vi "Actor Core.vi"(8 "error in":errorcluster, 11 "ExampleViewManager In":refnum<class "ExampleViewManager.lvclass">) -> (0 "error out":errorcluster, 3 "Actor out":refnum<class "Actor.lvclass">)   [LabVIEW 2017, in "MVA Example.lvlib" / "ExampleViewManager.lvclass"]
doc: "(<B>Filename</B>: Actor Framework.lvlib:Actor.lvclass:Actor Core.vi)\n\nReceives messages to the actor, reacts to them, and initiates any error handling that may shut the actor down.\n\nDescendant classes may override this VI to append parallel tasks for the actor to complete while it handles messages. Overrides use the Call Parent Method node.\n\n<License>\nCopyright © 2017 Composed Systems, LLC | All rights reserved\nwww.composed.io\n\nAuthor: Ethan Stern <ethan.stern@composed.io>\n\nThis software is provided \"AS IS\" WITHOUT WARRANTIES, either express or implied, AND IS FOR EDUCATIONAL PURPOSES ONLY.\n</License>MVA Framework 1.6.0.31\nEthan Stern - Composed Systems\nCopyright (c) 2018, Composed Systems"
uses:
  ExampleViewManager.lvclass
  C:/Program Files (x86)/National Instruments/LabVIEW 2017/vi.lib/Composed Systems/MVA Framework/Framework/ActorEvents/IEventAggregator/IEventAggregator.lvclass
  C:/Program Files (x86)/National Instruments/LabVIEW 2017/vi.lib/ActorFramework/Actor/Actor.lvclass
  <vilib>/ActorFramework/Actor/Actor.lvclass
  <vilib>/event_ctls.llb/lveventtype.ctl
  ExampleViewManager.lvclass/ExampleViewManager.ctl
  <vilib>/ActorFramework/Actor/Actor.lvclass/Actor.ctl
  <vilib>/ActorFramework/Message Enqueuer/Message Enqueuer.lvclass/Message Enqueuer.ctl
  <vilib>/ActorFramework/Report Error Msg/Report Error Msg.lvclass/Report Error Msg.ctl
  <vilib>/ActorFramework/Message Enqueuer/Init from Existing Queue.vi
  <vilib>/ActorFramework/Message Enqueuer/Enqueue.vi
  <vilib>/ActorFramework/Report Error Msg/Report Error Msg.lvclass
  C:/Program Files (x86)/National Instruments/LabVIEW 2017/vi.lib/ActorFramework/Message/Message.lvclass
  <vilib>/ActorFramework/Message Priority Queue/Priority Enqueue.vi
  <vilib>/ActorFramework/Message Enqueuer/Message Enqueuer.lvclass
  <vilib>/Composed Systems/MVA Framework/Framework/IViewManager/IViewManager/IViewManager.lvclass
  MenuButton/MenuButton.lvclass
  MenuButton Event Handler/MenuButton Event Handler.lvclass
  <vilib>/Composed Systems/MVA Framework/Framework/ActorEvents/IEventAggregator/IEventAggregator.lvclass
  <vilib>/Composed Systems/MVA Framework/Framework/IViewable/ProtectedSubpanel/ProtectedSubpanel.lvclass
panel:
  in  "Bool2":bool caption="Blank"
  in  "Main Menu 3":bool caption="Blank"
  in  "Chart2":bool caption="Blank"
  in  "Main Menu 2":bool caption="Blank"
  in  "Slide":bool caption="Blank"
  in  "Listbox":bool caption="Blank"
  in  "Bool1":bool caption="Blank"
  in  "Chart":bool caption="Blank"
  in  "Quad Menu":bool caption="Blank"
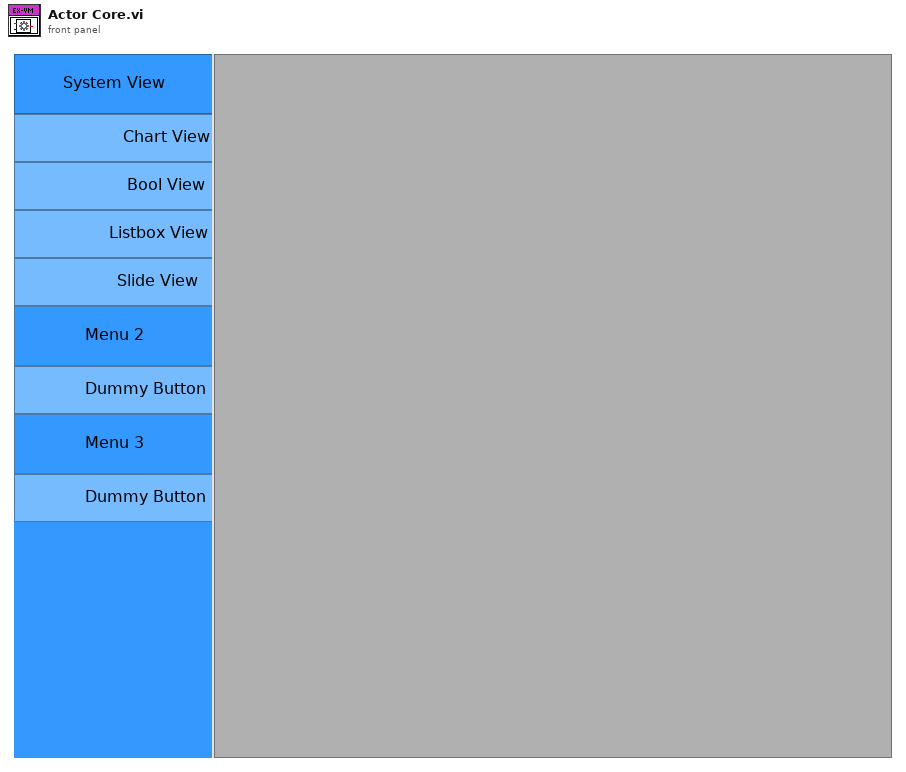
[diagram p1: front panel]
types:
  T1 = typedef "lveventtype.ctl" = enum32{"Null", "Timeout", "Annotation Menu Selection", "Annotation Menu Selection?", "App Instance Close", "App Instance Close?", "Autoscale Range Change", "Bookmark Info Change", "Cell Edit", "Cell Edit?", "Cursor Grab", "Cursor Grab?", "Cursor Menu Selection", "Cursor Menu Selection?", "Cursor Move", "Cursor Release", "Data Change", "Direction Change", "Display State Change", "Drag Ended", "Drag Enter", "Drag Leave", "Drag Over", "Drag Source Update", "Drag Starting", "Drag Starting?", "Drop", "Exec State Change", "Key Down", "Key Down?", "Key Repeat", "Key Repeat?", "Key Up", "Listbox Double Click", "Menu Activation?", "Menu Selection (App)", "Menu Selection? (App)", "Menu Selection (User)", "Mouse Down", "Mouse Down?", "Mouse Enter", "Mouse Leave", "Mouse Move", "Mouse Up", "Mouse Wheel", "NI Security User Change (App)", "Pane Size", "Panel Close", "Panel Close?", "Panel Resize", "Plot Attribute Change", "Scale Range Change", "Shortcut Menu Activation?", "Shortcut Menu Selection (App)", "Shortcut Menu Selection? (App)", "Shortcut Menu Selection (User)", "Tree Double Click", "Tree Drag", "Tree Drag?", "Tree Drop", "Tree Drop?", "Tree Item Close", "Tree Item Close?", "Tree Item Open", "Tree Item Open?", "User Event", "Value Change"}
  T2 = typedef "IViewable.lvlib/ProtectedSubpanel.lvclass/Protected Subpanel Reference.ctl" = refnum<data-value>
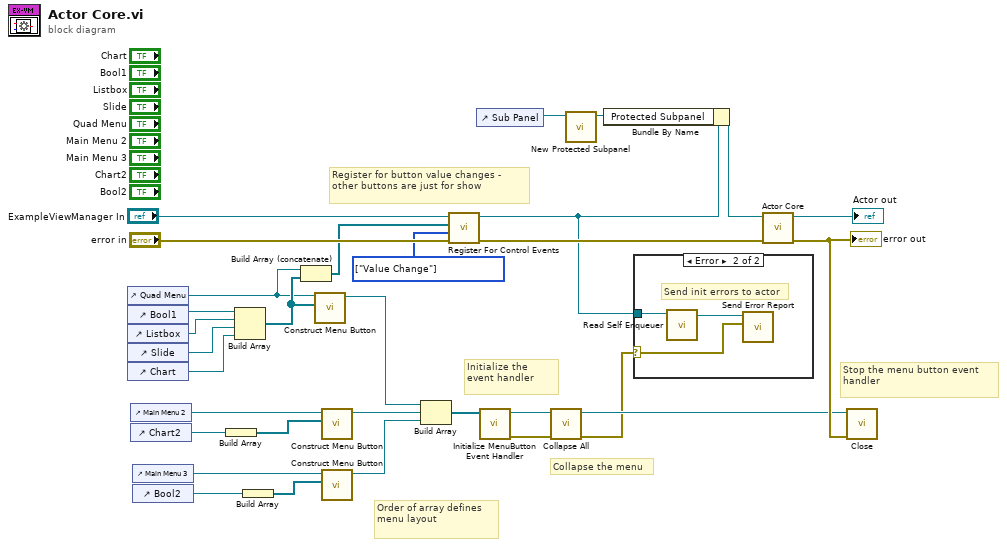
[diagram p0: block diagram]
diagram:
  w8 = T1[] [enum."Value Change"] items=["Null", "Timeout", "Annotation Menu Selection", "Annotation Menu Selection?", "App Instance Close", "App Instance Close?", "Autoscale Range Change", "Bookmark Info Change", "Cell Edit", "Cell Edit?", "Cursor Grab", "Cursor Grab?", "Cursor Menu Selection", "Cursor Menu Selection?", "Cursor Move", "Cursor Release", "Data Change", "Direction Change", "Display State Change", "Drag Ended", "Drag Enter", "Drag Leave", "Drag Over", "Drag Source Update", "Drag Starting", "Drag Starting?", "Drop", "Exec State Change", "Key Down", "Key Down?", "Key Repeat", "Key Repeat?", "Key Up", "Listbox Double Click", "Menu Activation?", "Menu Selection (App)", "Menu Selection? (App)", "Menu Selection (User)", "Mouse Down", "Mouse Down?", "Mouse Enter", "Mouse Leave", "Mouse Move", "Mouse Up", "Mouse Wheel", "NI Security User Change (App)", "Pane Size", "Panel Close", "Panel Close?", "Panel Resize", "Plot Attribute Change", "Scale Range Change", "Shortcut Menu Activation?", "Shortcut Menu Selection (App)", "Shortcut Menu Selection? (App)", "Shortcut Menu Selection (User)", "Tree Double Click", "Tree Drag", "Tree Drag?", "Tree Drop", "Tree Drop?", "Tree Item Close", "Tree Item Close?", "Tree Item Open", "Tree Item Open?", "User Event", "Value Change"] ("Registration Types")
  # "Collapse the menu"
  # "Order of array defines menu layout"
  # "Initialize the event handler"
  # "Stop the menu button event handler"
  # "Register for button value changes - other buttons are just for show"
  n1 = control-ref of="Quad Menu"() -> (w10:refnum<vi>)
  n2 = control-ref of="Bool1"() -> (w30:refnum<vi>)
  n3 = control-ref of="Listbox"() -> (w29:refnum<vi>)
  n4 = control-ref of="Slide"() -> (w28:refnum<vi>)
  n5 = control-ref of="Chart"() -> (w27:refnum<vi>)
  n6 = control-ref of="Main Menu 2"() -> (w25:refnum<vi>)
  n7 = control-ref of="Chart2"() -> (w26:refnum<vi>)
  n8 = control-ref of="Main Menu 3"() -> (w23:refnum<vi>)
  n9 = control-ref of="Bool2"() -> (w22:refnum<vi>)
  n10 = Build Array(w26) -> (w24:refnum<vi>[])
  n11 = Build Array(w30, w29, w28, w27) -> (w11:refnum<vi>[])
  n12 = Build Array(w22) -> (w6:refnum<vi>[])
  n13 = Build Array (concatenate)(w10, w11) -> (w9:refnum<vi>[])
  n14 = call "Construct Menu Button.vi"("Nested Item Refs"=w11, "Menu Reference"=w10) -> ("MenuButton out"=w21:refnum<class "MenuButton.lvclass">)  [unwired: 9 in]
  n15 = call "Construct Menu Button.vi"("Nested Item Refs"=w24, "Menu Reference"=w25) -> ("MenuButton out"=w20:refnum<class "MenuButton.lvclass">)  [unwired: 9 in]
  n16 = call "Construct Menu Button.vi"("Nested Item Refs"=w6, "Menu Reference"=w23) -> ("MenuButton out"=w19:refnum<class "MenuButton.lvclass">)  [unwired: 9 in]
  n17 = Build Array(w21, w20, w19) -> (w18:refnum<class "MenuButton.lvclass">[])
  n18 = call <vilib>:"Register For Control Events.vi"("error in (no error)"="error in", "Registration Types"=w8, "Control Refnums"=w9, "IEventAggregator In"="ExampleViewManager In") -> ("error out"=w4:errorcluster, "IEventAggregator Out"=w3:refnum<class "ExampleViewManager.lvclass">)  [unwired: 6 in]
  n19 = control-ref of="Sub Panel"() -> (w5:refnum<vi>)
  n20 = call "Initialize MenuButton Event Handler.vi"("Menu Buttons"=w18) -> ("error out"=w16:errorcluster, "MenuButton Event Handler out"=w17:refnum<class "MenuButton Event Handler.lvclass">)  [unwired: 9 in]
  n21 = call "Collapse All.vi"("error in (no error)"=w16, "MenuButton Event Handler in"=w17) -> ("error out"=w7:errorcluster, "MenuButton Event Handler out"=w14:refnum<class "MenuButton Event Handler.lvclass">)  [unwired: 8 in]
  n22 = call <vilib>:"New Protected Subpanel.vi"("SubPnl Refnum"=w5) -> ("Protected Subpanel"=w2:T2)  [unwired: 9 in, 1 out]
  n23 = Bundle By Name(cluster=w3, "Protected Subpanel"=w2) -> (w1:refnum<class "ExampleViewManager.lvclass">)
  n24 = case shown="Error" w7 {
    selector: w7 -> [_ w33]
    tunnel: w3 -> [_ w32]
    frame No Error {
    }
    frame Error {
      # "Send init errors to actor"
      n25 = call <vilib>:"Read Self Enqueuer.vi"("Actor"=w32) -> ("Self Enqueuer"=w34:refnum<class "Message Enqueuer.lvclass">)  [unwired: 10 in]
      n26 = call <vilib>:"Send Error Report.vi"("Error From Sender"=w33, "Message Enqueuer"=w34) -> ()  [unwired: 9 in, 1 out]
    }
  }
  n27 = call-parent "Actor Core.vi"("error in"=w4, "IViewable In"=w1) -> ("error out"=w15:errorcluster, "Actor out"=→"Actor out":refnum<class "Actor.lvclass">)  [unwired: 8 in]
  "error out" <- w15
  n28 = call "Close.vi"("error in (no error)"=w15, "MenuButton Event Handler in"=w14) -> ()  [unwired: 9 in, 1 out]
